vi "Actor Core.vi"(8 "error in":errorcluster, 11 "Example Controller":refnum<class "Example Controller Actor.lvclass">) -> (0 "error out":errorcluster, 3 "Actor out":refnum<class "Actor.lvclass">)   [LabVIEW 2017, in "Example Controller Actor.lvlib" / "Example Controller Actor.lvclass"]
doc: "This is Actor Core.vi, the main message handling loop for Actors. An actor usually just sits in this loop and processes messages as they arrive. Any error returned by the message Do.vi call will stop the loop, with error code 43 as the cannonical signal to stop with no error sent to caller. Descendants may override that in Handle Error.vi."
uses:
  Example Controller Actor.lvclass
  C:/Projects/Shared Libraries/Event Actors/Controller Actor/Controller Actor.lvclass
  C:/Program Files/National Instruments/LabVIEW 2017/vi.lib/ActorFramework/Actor/Actor.lvclass
  <vilib>/ActorFramework/Actor/Actor.lvclass
  Registered Views.ctl
  Controller Actor/View Settings.ctl
  Example Controller Actor.lvclass/Example Controller Actor.ctl
  Controller Actor/Controller Actor.lvclass/Controller Actor.ctl
  <vilib>/ActorFramework/Actor/Actor.lvclass/Actor.ctl
  <vilib>/ActorFramework/Message Enqueuer/Message Enqueuer.lvclass/Message Enqueuer.ctl
  Example Events/Timestamp Event.lvclass
  C:/Projects/Shared Libraries/Event Actors/Event/Event.lvclass
  Event/Event.lvclass/Event.ctl
  Example View Actor/Example View Actor Messages/Update Time Event Msg/Update Time Event Msg.lvclass
  C:/Projects/Shared Libraries/Event Actors/Event Handlers/Abstract Event Message for View/Abstract Event Message for View.lvclass
  Example Events/Double Array Event.lvclass
  Example View Actor/Example View Actor Messages/Update Array Event Msg/Update Array Event Msg.lvclass
  Write Boolean Notifier.vi
  Controller Actor/properties/Read Registered Views Event Ref.vi
  Controller Actor/properties/Read View Settings Event Ref.vi
  <vilib>/ActorFramework/Message Enqueuer/Init from Existing Queue.vi
  <vilib>/ActorFramework/Message Enqueuer/Enqueue.vi
  <vilib>/ActorFramework/Stop Msg/Stop Msg.lvclass
  C:/Program Files/National Instruments/LabVIEW 2017/vi.lib/ActorFramework/Message/Message.lvclass
  <vilib>/Utility/LVClass/Get LV Class Name.vi
  <resource>/AFDebug/Generate Trace for Message.vi
  <vilib>/ActorFramework/Message Priority Queue/Priority Enqueue.vi
  <vilib>/ActorFramework/Message Enqueuer/Message Enqueuer.lvclass
  Timed Loop Controller/Timed Loop Controller/Timed Loop Controller.lvclass
  Event/Event.lvclass
  Controller Actor Messages/Register by Name Msg/Register by Name Msg.lvclass
  Controller Actor Messages/Unregister by Name Msg/Unregister by Name Msg.lvclass
  Controller Actor/Controller Actor.lvclass
  Controller Actor Messages/Read Registered Views Msg/Read Registered Views Msg.lvclass
  Controller Actor Messages/Read View Settings Msg/Read View Settings Msg.lvclass
  Controller Actor Messages/Write View Settings Msg/Write View Settings Msg.lvclass
panel:
  in  "View Settings":T1
  in  "Write View Settings":bool
  in  "Read View Settings":bool
  out "View Settings Read":T1
  in  "View":T2
  out "Boolean Chart":i16(graph)
  in  "Registered for Data":bool=TRUE
  in  "Registered for Time":bool=TRUE
  in  "Stop Button":bool
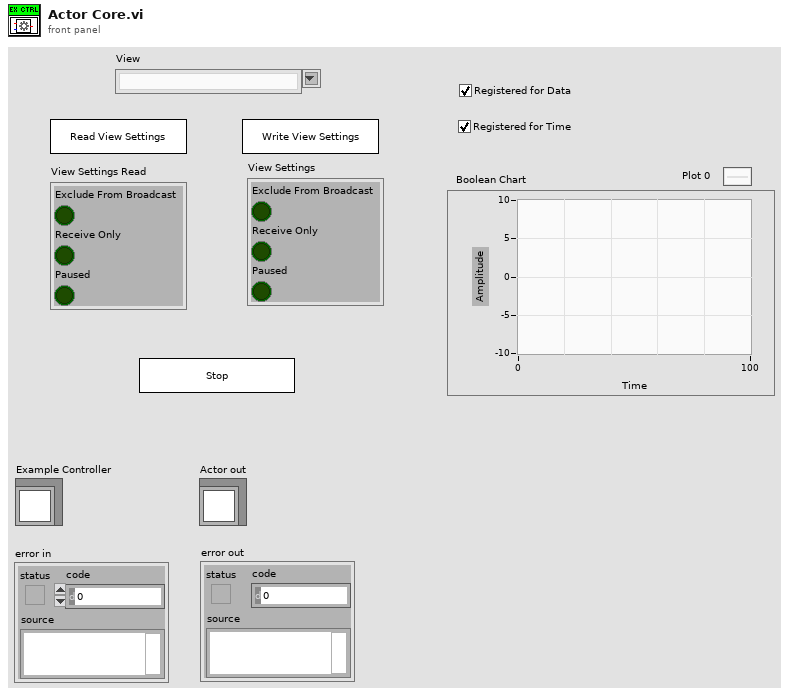
[diagram p1: front panel]
types:
  T1 = typedef "Event Actors.lvlib/Controller Actor.lvclass/View Settings.ctl" = cluster{"Exclude From Broadcast":bool, "Receive Only":bool, "Paused":bool}
  T2 = typedef "Example Controller Actor.lvlib/Example Controller Actor.lvclass/Registered Views.ctl" = string
  T3 = typedef "Event Actors.lvlib/Controller Actor.lvclass/Registered Views Event Ref.ctl" = refnum<user-event>
  T4 = typedef "Event Actors.lvlib/Controller Actor.lvclass/View Settings Event Ref.ctl" = refnum<user-event>
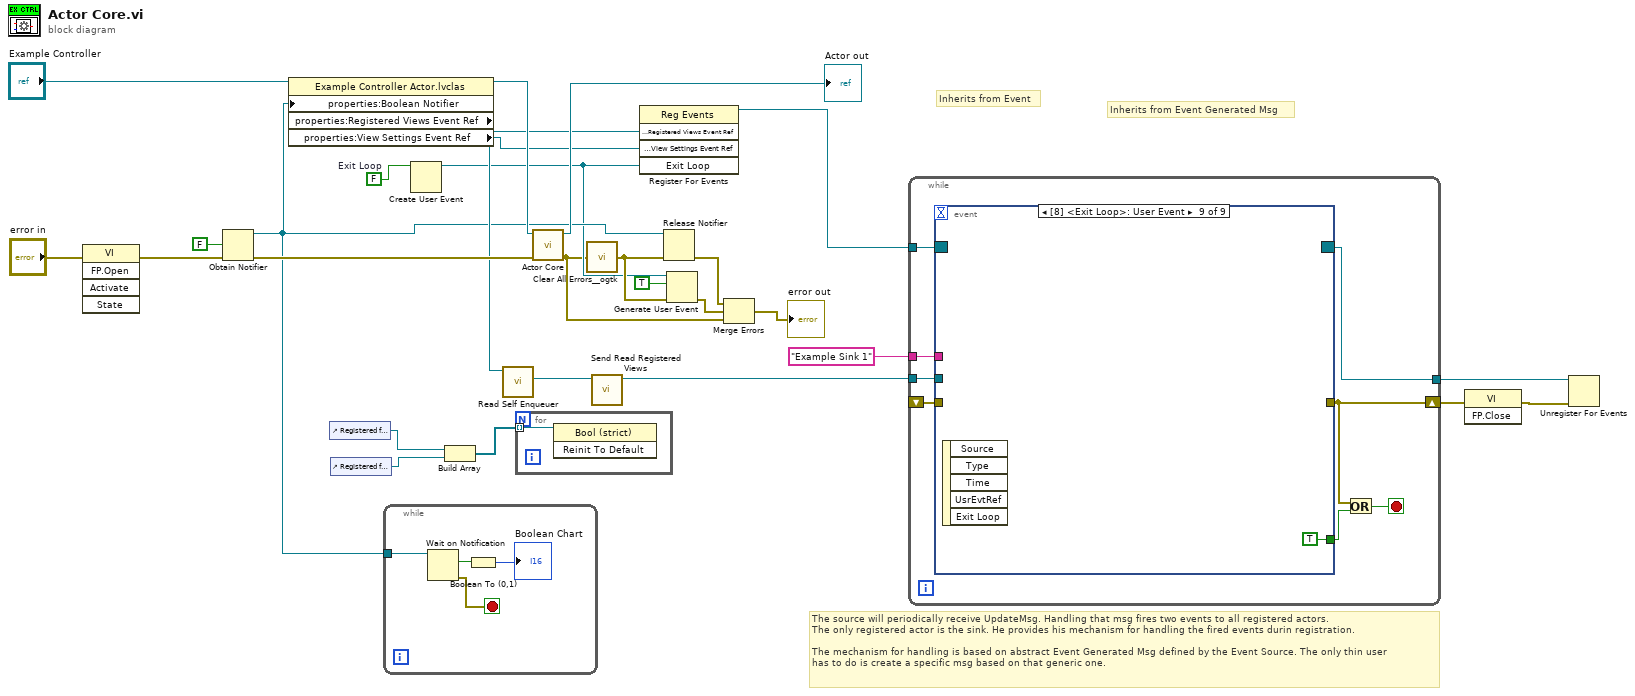
[diagram p0: block diagram]
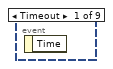
[diagram p2: hidden frame]
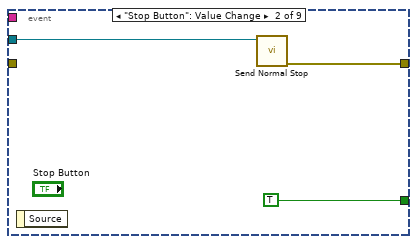
[diagram p3: hidden frame]
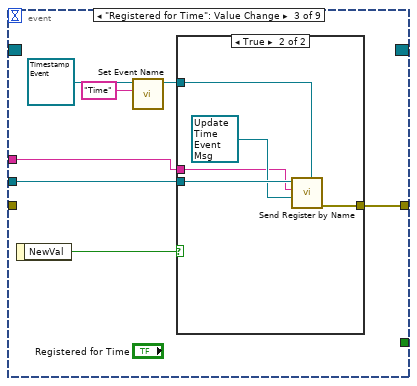
[diagram p4: hidden frame]
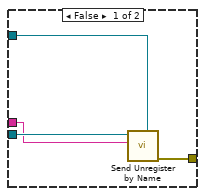
[diagram p5: hidden frame]
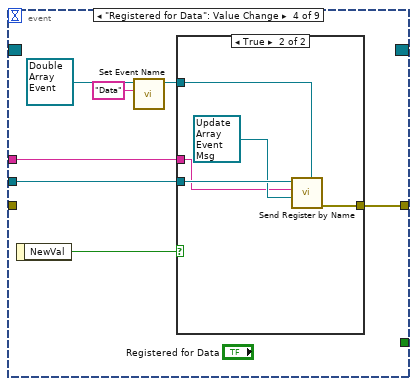
[diagram p6: hidden frame]
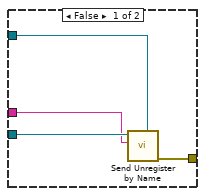
[diagram p7: hidden frame]
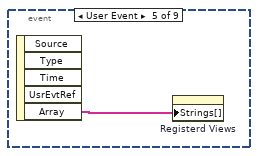
[diagram p8: hidden frame]
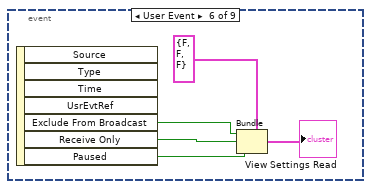
[diagram p9: hidden frame]
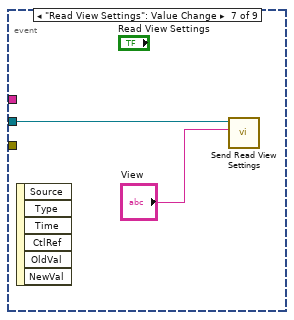
[diagram p10: hidden frame]
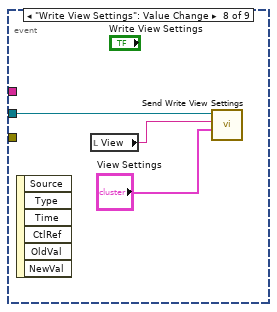
[diagram p11: hidden frame]
diagram:
  w10 = FALSE  # Exit Loop
  # "The source will periodically receive UpdateMsg. Handling that msg fires two events to all registered actors.\nThe only registered actor is the sink. He provides his mechanism for handling the fired events durin registration.\n\nThe mechanism for handling is based on abstract Event Generated Msg defined by the Event Source. The only thin user\nhas to do is create a specific msg based on that generic one."
  # "Inherits from Event"
  # "Inherits from Event Generated Msg"
  n1 = invoke on="Invoke Node" class="VI" method="FP.Open"(error in="error in") -> (error out=w1:errorcluster)  [unwired: 4 in, 4 out]
  n2 = Obtain Notifier(notification data type=FALSE, error in (no error)=w1) -> (notifier out=w18:refnum<notifier>, error out=w20:errorcluster)  [unwired: 2 in, 1 out]
  n3 = property class="Example Controller Actor.lvclas"(reference="Example Controller", "properties:Boolean Notifier"=w18) -> (reference out=w19:refnum<class "Example Controller Actor.lvclass">, "properties:Registered Views Event Ref"=w17:T3, "properties:View Settings Event Ref"=w16:T4)  [unwired: 1 in, 1 out]
  n4 = control-ref of="Registered for Time"() -> (w24:refnum<vi>)
  n5 = control-ref of="Registered for Data"() -> (w23:refnum<vi>)
  n6 = while {
    tunnel: w18 -> [w32]
    stop <- w29 stop-if-true
    n7 = Wait on Notification(notifier=w32) -> (notification=w31:bool, error out=w29:errorcluster)  [unwired: 3 in, 2 out]
    n8 = Boolean To (0,1)(Boolean=w31) -> (0, 1=→"Boolean Chart":i16)
  }
  n9 = Create User Event(user event datatype=w10) -> (user event=w7:refnum<user-event>)  [unwired: 1 in, 1 out]
  n10 = Build Array(w24, w23) -> (w22:refnum<vi>[])
  n11 = call <vilib>:"Read Self Enqueuer.vi"("Actor"=w19) -> ("Self Enqueuer"=w12:refnum<class "Message Enqueuer.lvclass">)  [unwired: 10 in]
  n12 = for {
    tunnel: w22 -> [w33] mode=indexing
    n13 = invoke class="Bool (strict)" method="Reinit To Default"(reference=w33) -> ()  [unwired: 2 in, 3 out]
  }
  n14 = call-parent "Actor Core.vi"("error in"=w20, "Timed Loop Controller"=w19) -> ("error out"=w4:errorcluster, "Actor out"=→"Actor out":refnum<class "Actor.lvclass">)  [unwired: 8 in]
  n15 = call <userlib>:"Clear All Errors__ogtk.vi"("Error In"=w4) -> ("Error Out"=w8:errorcluster)  [unwired: 3 in]
  n16 = call "Send Read Registered Views.vi"("Message Enqueuer in"=w12) -> ("Message Enqueuer out"=w11:refnum<class "Message Enqueuer.lvclass">)  [unwired: 9 in, 1 out]
  n17 = register-events(w17, w16, w7) -> (reference out=w15:refnum<event-registration>)  [unwired: 2 in, 1 out]
  n18 = Release Notifier(notifier=w18, error in (no error)=w8) -> (error out=w6:errorcluster)  [unwired: 1 in, 2 out]
  n19 = Generate User Event(user event=w7, event data cluster=TRUE ("event data"), error in=w8) -> (error out=w5:errorcluster)  [unwired: 1 in, 1 out]
  n20 = Merge Errors(w6, w5, w4) -> (→"error out":errorcluster)
  n21 = while {
    tunnel: w11 -> [w40]
    shift-right: [w38] -> w27
    shift-left: _ -> [w41]
    tunnel: "Example Sink 1" ("Debug Alias") -> [w36]
    tunnel: w15 -> [w35]
    tunnel: [w34] -> w13
    stop <- w37 stop-if-true
    n22 = event shown="[8] <Exit Loop>: User Event" {
      selector: w35 -> [_ _ _ _ _ _ _ _ _]
      dyn-events: [_ _ _ _ _ _ _ _ _] -> w34
      timeout: _ -> [_ _ _ _ _ _ _ _ _]
      tunnel: w41 -> [_ _ _ _ _ _ _ _ _]
      tunnel: w40 -> [_ w43 w50 w66 _ _ w83 w85 _]
      tunnel: [_ w44 w49 w65 _ _ _ _ _] -> w38
      tunnel: [_ TRUE _ _ _ _ _ _ TRUE] -> w39
      tunnel: w36 -> [_ _ w45 w61 _ _ _ _ _]
      event Timeout {
        n23 = event-data() -> ()  [unwired: 1 in, 1 out]
      }
      event "Stop Button": Value Change {
        n24 = event-data() -> ()  [unwired: 1 in, 1 out]
        n25 = call <vilib>:"Send Normal Stop.vi"("Message Enqueuer"=w43) -> ("error out"=w44:errorcluster)  [unwired: 10 in]
      }
      event "Registered for Time": Value Change {
        n26 = event-data() -> ("NewVal"=w51:bool)  [unwired: 1 in]
        n27 = call "Set Event Name.vi"("Name (Generic)"="Time", "Event In"=refnum<class "Timestamp Event.lvclass"> refnum ("Timestamp Event.lvclass")) -> ("Event Out"=w46:refnum<class "Timestamp Event.lvclass">)  [unwired: 9 in]
        n28 = case shown="True" w51 {
          tunnel: w50 -> [w55 w60]
          tunnel: w46 -> [w54 w58]
          tunnel: [w53 w57] -> w49
          tunnel: w45 -> [w52 w56]
          frame False {
            n29 = call "Send Unregister by Name.vi"("Event"=w54, "View Name"=w52, "Message Enqueuer in"=w55) -> ("error out"=w53:errorcluster)  [unwired: 7 in, 1 out]
          }
          frame True {
            n30 = call "Send Register by Name.vi"("Event"=w58, "Event Fire Handler"=refnum<class "Update Time Event Msg.lvclass"> refnum ("Update Time Msg.lvclass"), "View Name"=w56, "Message Enqueuer in"=w60) -> ("error out"=w57:errorcluster)  [unwired: 6 in, 1 out]
          }
        }
      }
      event "Registered for Data": Value Change {
        n31 = event-data() -> ("NewVal"=w67:bool)  [unwired: 1 in]
        n32 = call "Set Event Name.vi"("Name (Generic)"="Data", "Event In"=refnum<class "Double Array Event.lvclass"> refnum ("Double Array Event.lvclass")) -> ("Event Out"=w63:refnum<class "Double Array Event.lvclass">)  [unwired: 9 in]
        n33 = case shown="True" w67 {
          tunnel: w66 -> [w71 w76]
          tunnel: w63 -> [w70 w75]
          tunnel: [w69 w74] -> w65
          tunnel: w61 -> [w68 w72]
          frame False {
            n34 = call "Send Unregister by Name.vi"("Event"=w70, "View Name"=w68, "Message Enqueuer in"=w71) -> ("error out"=w69:errorcluster)  [unwired: 7 in, 1 out]
          }
          frame True {
            n35 = call "Send Register by Name.vi"("Event"=w75, "Event Fire Handler"=refnum<class "Update Array Event Msg.lvclass"> refnum ("Update Array Msg.lvclass"), "View Name"=w72, "Message Enqueuer in"=w76) -> ("error out"=w74:errorcluster)  [unwired: 6 in, 1 out]
          }
        }
      }
      event User Event {
        n36 = event-data() -> ("Array"=w77:string[])  [unwired: 1 in, 4 out]
        n37 = property on="Registerd Views" class="CmbBox (strict)"("Strings[]"=w77) -> ()  [unwired: 2 in, 2 out]
      }
      event User Event {
        n38 = event-data() -> ("Exclude From Broadcast"=w81:bool, "Receive Only"=w80:bool, "Paused"=w79:bool)  [unwired: 1 in, 4 out]
        n39 = Bundle(cluster=T1 {"Exclude From Broadcast"=FALSE, "Receive Only"=FALSE, "Paused"=FALSE} ("Sink Settings"), "Exclude From Broadcast"=w81, "Receive Only"=w80, "Paused"=w79) -> (→"View Settings Read":T1)
      }
      event "Read View Settings": Value Change {
        n40 = event-data() -> ()  [unwired: 1 in, 6 out]
        n41 = call "Send Read View Settings.vi"("View Name"="View", "Message Enqueuer in"=w83) -> ()  [unwired: 8 in, 2 out]
      }
      event "Write View Settings": Value Change {
        n42 = event-data() -> ()  [unwired: 1 in, 6 out]
        n43 = local read "View"() -> (w86:T2)
        n44 = call "Send Write View Settings.vi"("View Settings"="View Settings", "View Name"=w86, "Message Enqueuer in"=w85) -> ()  [unwired: 7 in, 2 out]
      }
      event User Event {
        n45 = event-data() -> ()  [unwired: 1 in, 5 out]
      }
    }
    n46 = Or(x=w38, y=w39) -> (x .or. y?=w37:bool)
  }
  n47 = invoke class="VI" method="FP.Close"(error in=w27) -> (error out=w14:errorcluster)  [unwired: 2 in, 2 out]
  n48 = Unregister For Events(event registration refnum=w13, error in=w14) -> ()  [unwired: 1 out]
